vi "ProjectCode_WithoutHardware.vi"() -> ()   [LabVIEW 2023]
panel:
  in  "Plant Name":string
  in  "Recipient Email Address:":string
  out "Analog Data":dbl(graph)
  out "Time remaining (sec)":i32
  in  "Duration (HOUR[s])":dbl
  out "Time Elapsed (sec)":i32
  in  "Duration (MIN[s])":dbl
  in  "Yes/No":bool
  out "Sensor Output:":dbl
  in  "stop":bool
  out "Plamt Status":T1(ring)
  out "Need to Water?":bool
  # "Email:"
  # "Arduino Parameters:"
  # "<-- Seperate multiple recipients with comma"
  # "Send Additional email reminders?"
  # "How Long to Send Reminder:"
  # "Troubleshooting:"
  # "Reminder Time:"
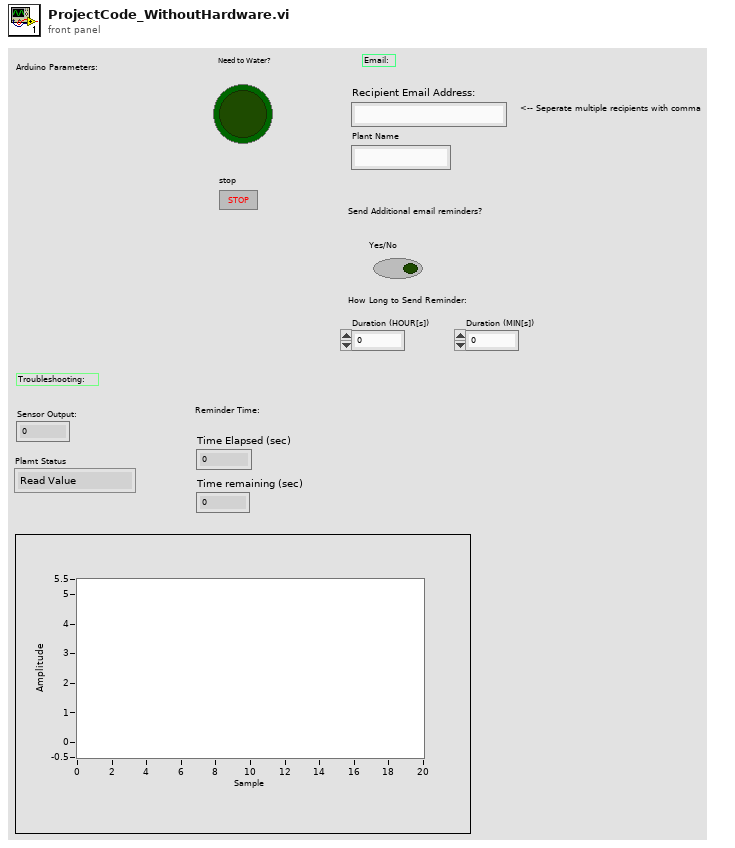
[diagram p1: front panel]
types:
  T1 = enum16{"Read Value", "Send Reminder", "Reminder Timer", "Button Fallbaack"}
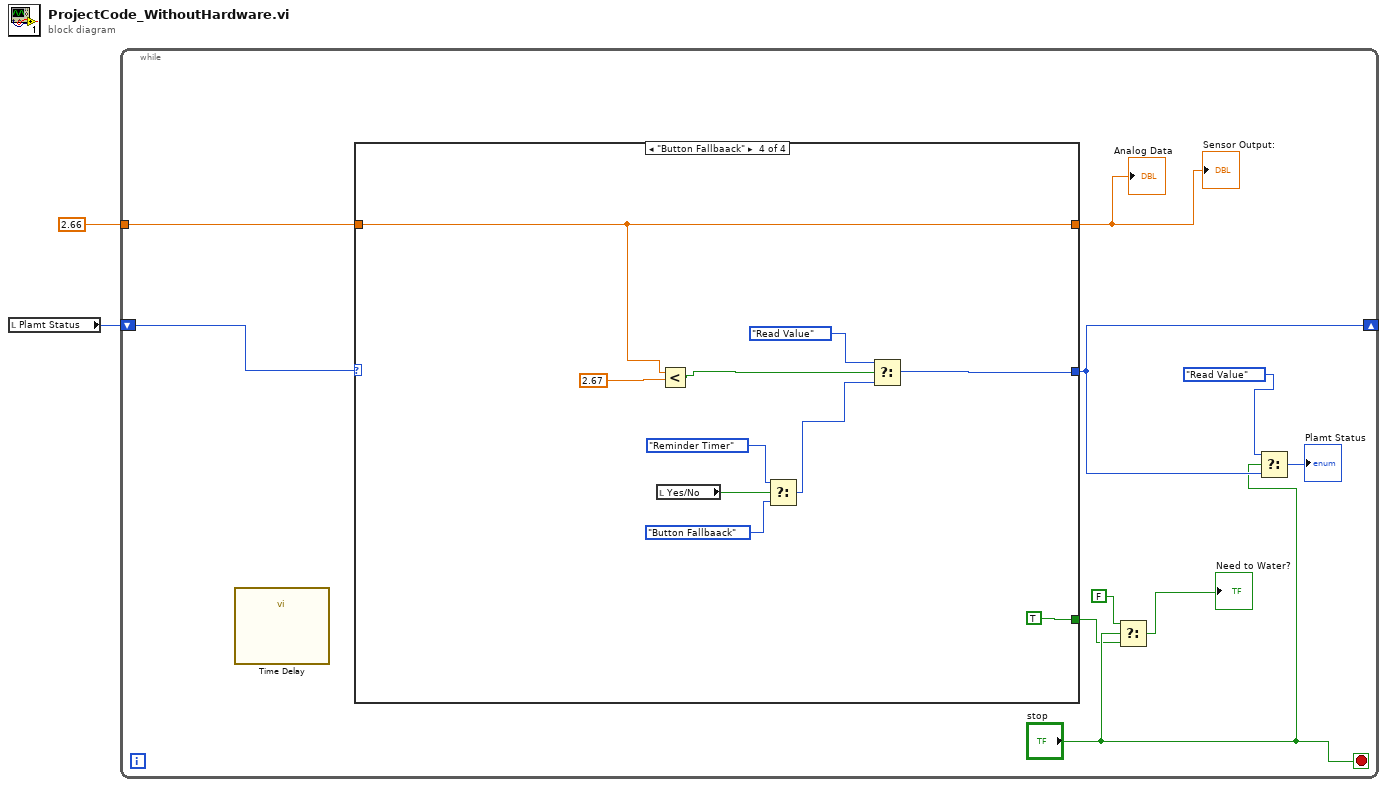
[diagram p0: block diagram]
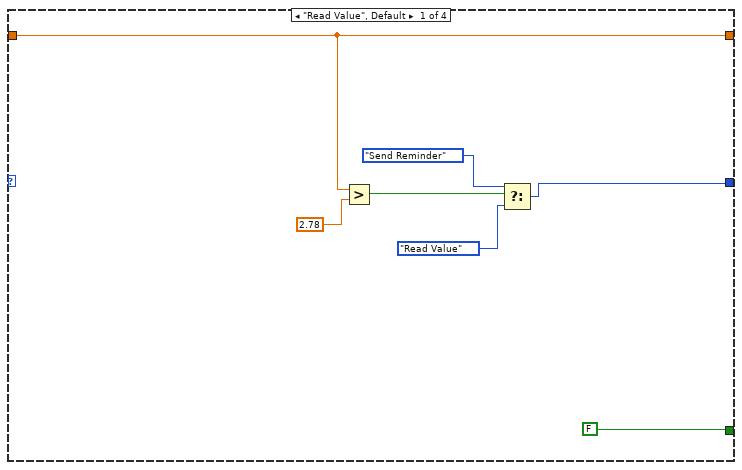
[diagram p2: hidden frame]
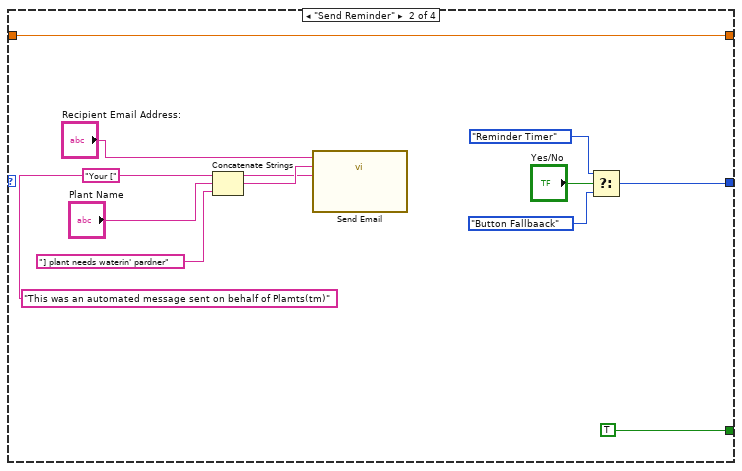
[diagram p3: hidden frame]
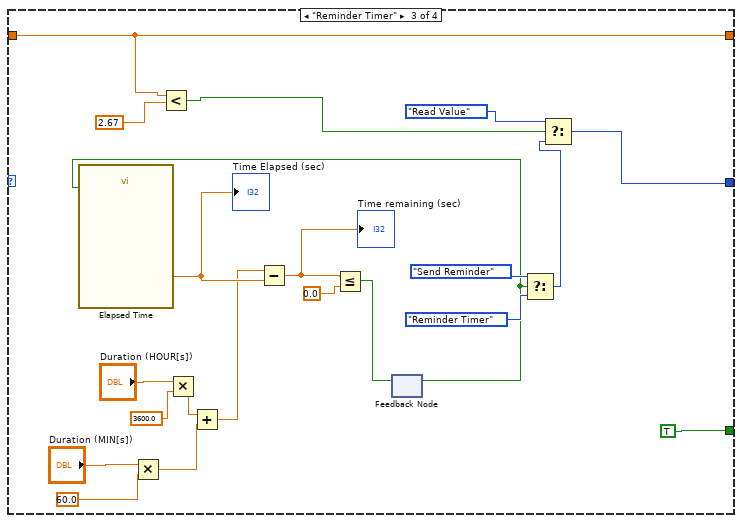
[diagram p4: hidden frame]
diagram:
  n1 = local read "Plamt Status"() -> (w2:T1)
  n2 = while {
    shift-right: [w11] -> _
    shift-left: w2 -> [w10]
    tunnel: 2.66 -> [w7]
    stop <- "stop" stop-if-true
    n3 = call "Time Delay"() -> ()  [unwired: 11 in, 1 out]
    n4 = case shown="\"Button Fallbaack\"" w10 {
      tunnel: w7 -> [w15 w30 w34 w54]
      tunnel: [w17 w29 w39 w61] -> w11
      tunnel: [FALSE TRUE TRUE TRUE] -> w4
      tunnel: [w15 w30 w34 w54] -> w8
      frame "Read Value", Default {
        n5 = Greater?(x=w15, y=2.78) -> (0:w18:bool)
        n6 = Select(t=T1."Send Reminder" ("Plamt Status"), s=w18, f=T1."Read Value" ("Plamt Status")) -> (s? t:f=w17:T1)
      }
      frame "Send Reminder" {
        n7 = Concatenate Strings("Your [", "Plant Name", "] plant needs waterin' pardner") -> (w25:string)
        n8 = call "Send Email"("Message"="This was an automated message sent on behalf of Plamts(tm)", "Subject"=w25, "Recipients"="Recipient Email Address:") -> ()  [unwired: 8 in, 1 out]
        n9 = Select(t=T1."Reminder Timer" ("Plamt Status"), s="Yes/No", f=T1."Button Fallbaack" ("Plamt Status")) -> (s? t:f=w29:T1)
      }
      frame "Reminder Timer" {
        n10 = Multiply(x="Duration (MIN[s])", y=60.0) -> (x*y=w45:dbl)
        n11 = Less?(x=w34, y=2.67) -> (x < y?=w32:bool)
        n12 = Multiply(x="Duration (HOUR[s])", y=3600.0) -> (x*y=w50:dbl)
        n13 = Add(x=w50, y=w45) -> (x+y=w51:dbl)
        n14 = feedback #1() -> (w38:bool)  [unwired: 1 in]
        n15 = call "Elapsed Time"("Reset"=w38) -> ("Elapsed Time (s)"=w52:dbl)  [unwired: 11 in, 7 out]
        "Time Elapsed (sec)" <- w52
        n16 = Subtract(x=w51, y=w52) -> (x-y=w36:dbl)
        "Time remaining (sec)" <- w36
        n17 = Less Or Equal?(x=w36, y=0.0) -> (x <= y?=w35:bool)
        n18 = feedback-in #1(w35) -> ()
        n19 = Select(t=T1."Send Reminder" ("Plamt Status"), s=w38, f=T1."Reminder Timer" ("Plamt Status")) -> (s? t:f=w41:T1)
        n20 = Select(t=T1."Read Value" ("Plamt Status"), s=w32, f=w41) -> (s? t:f=w39:T1)
      }
      frame "Button Fallbaack" {
        n21 = local read "Yes/No"() -> (w56:bool)
        n22 = Less?(x=w54, y=2.67) -> (x < y?=w53:bool)
        n23 = Select(t=T1."Reminder Timer" ("Plamt Status"), s=w56, f=T1."Button Fallbaack" ("Plamt Status")) -> (s? t:f=w57:T1)
        n24 = Select(t=T1."Read Value" ("Plamt Status"), s=w53, f=w57) -> (s? t:f=w61:T1)
      }
    }
    "Sensor Output:" <- w8
    "Analog Data" <- w8
    n25 = Select(t=FALSE, s="stop", f=w4) -> (s? t:f=→"Need to Water?":bool)
    n26 = Select(t=T1."Read Value" ("Plamt Status"), s="stop", f=w11) -> (s? t:f=→"Plamt Status":T1)
  }
